vi "GenerateTemperaturePlots.vi"(11 "Temp Out":dbl[](array[numeric])) -> (2 "mean":dbl, 3 "Cluster":cluster{i32[], "Temp Out":dbl[]})   [LabVIEW 2018]
uses:
  <vilib>/Analysis/baseanly.llb/Mean (DBL).vi
  <vilib>/Analysis/NI_AALBase.lvlib
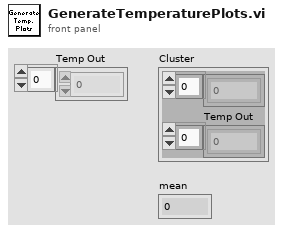
[diagram p1: front panel]
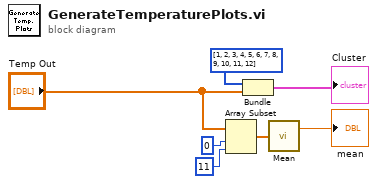
[diagram p0: block diagram]
diagram:
  n1 = Array Subset(array="Temp Out", index=0, length=11) -> (w3:dbl[])
  n2 = Bundle(i32[] [1, 2, 3, 4, 5, 6, 7, 8, 9, 10, 11, 12], "Temp Out"="Temp Out") -> (→"Cluster":cluster{i32[], "Temp Out":dbl[]})  [unwired: 1 in]
  n3 = call-poly <vilib>:"Mean.vi"("X"=w3) -> ("mean"=→"mean":dbl)  [unwired: 1 out]
